vi "connect.vi"(8 "error in (no error)":errorcluster, 9 "TCP_IP.lvclass (in)":refnum<class "TCP_IP.lvclass">, 11 "port":u16=9000) -> (0 "error out":errorcluster, 1 "TCP_IP.lvclass":refnum<class "TCP_IP.lvclass">)   [LabVIEW 2013, in "TCP_IP.lvclass"]
uses:
  TCP_IP.lvclass
  Experiment/states.ctl
  TCP_IP.lvclass/TCP_IP.ctl
  Experiment/Globals.vi
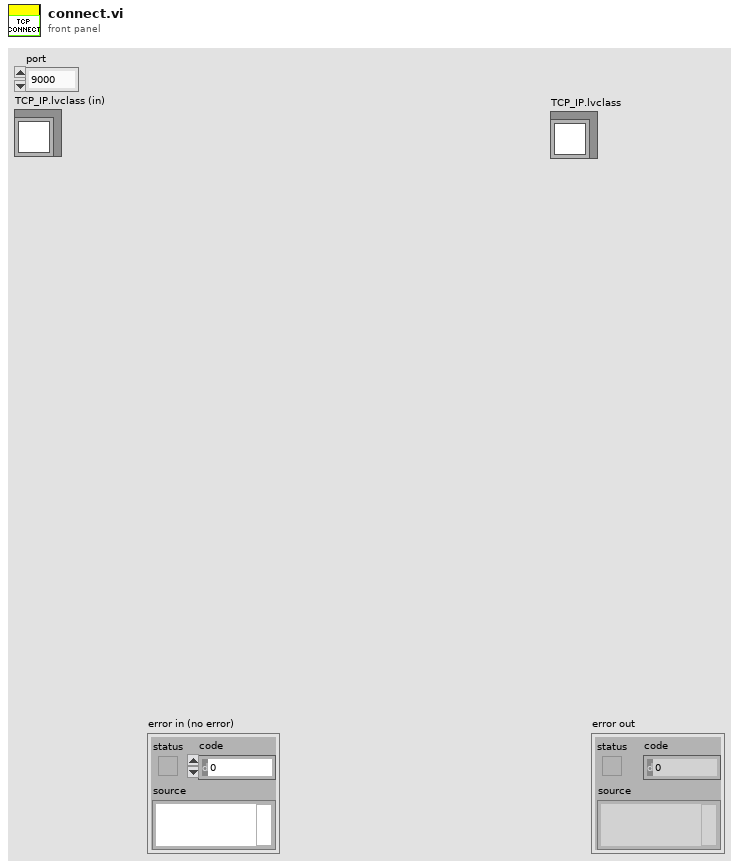
[diagram p1: front panel]
types:
  T1 = typedef "states.ctl" = enum16{"run", "pause", "shutdown gracefully", "halt immediately", "waiting for connection", "waiting for command"}
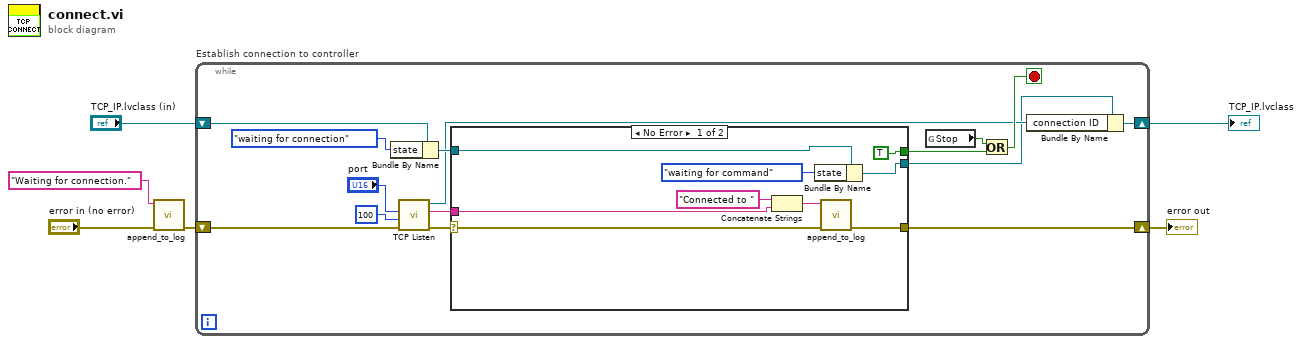
[diagram p0: block diagram]
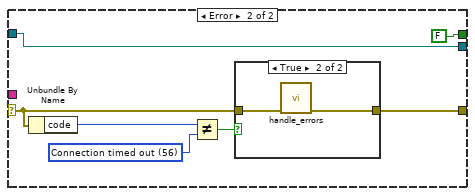
[diagram p2: hidden frame]
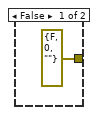
[diagram p3: hidden frame]
diagram:
  n1 = call "append_to_log.vi"("error in"="error in (no error)", "string"="Waiting for connection." ("Status")) -> ("error out"=w1:errorcluster)  [unwired: 9 in]
  n2 = while "Establish connection to controller" {
    shift-right: [w10] -> w5
    shift-left: "TCP_IP.lvclass (in)" -> [w14]
    shift-right: [w9] -> w4
    shift-left: w1 -> [w8]
    stop <- w16 stop-if-true
    n3 = Bundle By Name(cluster=w14, "state"=states."waiting for connection") -> (w13:refnum<class "TCP_IP.lvclass">)
    n4 = call <vilib>:"TCP Listen.vi"("error in (no error)"=w8, "timeout ms (wait forever: -1)"=100, "port"="port") -> ("error out"=w19:errorcluster, "remote address"=w20:string, "connection ID"=w12:refnum<k5>)  [unwired: 4 in, 2 out]
    n5 = case shown="No Error" w19 {
      selector: w19 -> [w26 w34]
      tunnel: w20 -> [w29 _]
      tunnel: [TRUE FALSE] -> w17
      tunnel: w13 -> [w24 w32]
      tunnel: [w23 w32] -> w11
      tunnel: [w22 w31] -> w9
      frame No Error {
        n6 = Concatenate Strings("Connected to " ("string"), w29) -> (w28:string)
        n7 = Bundle By Name(cluster=w24, "state"=states."waiting for command") -> (w23:refnum<class "TCP_IP.lvclass">)
        n8 = call "append_to_log.vi"("error in"=w26, "string"=w28) -> ("error out"=w22:errorcluster)  [unwired: 9 in]
      }
      frame Error {
        w37 = 56 items=["No Error", "Argument Error", "Memory Full", "Out of Zone", "End of File", "File Already Open", "Generic File IO Error", "File Not Found", "File Permission Error", "Disk Full", "Duplicate Path", "Too Many Files Open", "Not Enabled", "Resource File Not Found", "Cannot Add Resource", "Resource Not Found", "Image Not Found", "Image Memory Error", "Pen Does Not Exist", "Config Bad Type", "Config Token Not Found", "Config Parse Error", "Config Memory Error", "Bad External Code Format", "Bad External Code Offset", "External Code Not Present", "Null Window", "Destroy Window Mixup", "Null Menu", "Print Aborted", "Bad Print Record", "Print Driver Error", "Windows Error During Print", "Memory Error During Print", "Print Dialog Error", "Generic Print Error", "Invalid Device Refnum", "Device Not Found", "Device Parameter Error", "Device Unit Error", "Can't Open Device", "Device Call Aborted", "Generic Error", "Cancelled By User", "Object ID Too Low", "Object ID Too High", "Object Not In Heap", "Unknown Heap", "Bad DefProc ID", "DefProc Not In Table", "Message Out Of Range", "Null Method", "Unknown Message", "Manager Call Not Supported", "Bad address", "Connection In progress", "Connection timed out", "Connection is already in progress", "Network attribute not supported", "Network error", "Address in use", "System out of memory", "Connection aborted", "Connection refused", "Connection is not connected", "Connection is already connected", "Connection closed", "Initialize error (interapplication manager)", "Bad occurrence", "Wait on unbound occurrence handler", "Occurrence queue overflow", "Bad path", "Semaphore not signaled", "Unrecognized type (interapplication manager)"] ("1st Error to Convert")
        n9 = Unbundle By Name(w34) -> ("code"=w36:i32)
        n10 = Not Equal?(x=w36, y=w37) -> (x != y?=w35:bool)
        n11 = case shown="True" w35 {
          tunnel: w34 -> [_ w40]
          tunnel: [errorcluster {"status"=FALSE, "code"=0, "source"=""} ("error out") w39] -> w31
          frame False {
          }
          frame True {
            n12 = call "handle_errors.vi"("error in (no error)"=w40) -> ("error out"=w39:errorcluster)  [unwired: 14 in]
          }
        }
      }
    }
    n13 = global read "Globals.vi" "Stop"() -> (w7:bool)
    n14 = Or(x=w7, y=w17) -> (x .or. y?=w16:bool)
    n15 = Bundle By Name(cluster=w11, "connection ID"=w12) -> (w10:refnum<class "TCP_IP.lvclass">)
  }
  "TCP_IP.lvclass" <- w5
  "error out" <- w4
